vi "Set DeviceData_Status_IO.vi"(8 "error in (no error)":errorcluster, 9 "Trigger Event?":bool, 10 "Device Data":variant=variant(cluster{"DeviceName":string, "COM":refnum<visa-resource-name>, "Status String":string, "Input String":string, "DI Value ":i32}[] []), 11 "IO in":refnum<class "IO.lvclass">) -> (0 "error out":errorcluster, 3 "IO out":refnum<class "IO.lvclass">)   [LabVIEW 2022 SP3, in "IO.lvclass"]
uses:
  IO.lvclass
  IO.lvclass/IO.ctl
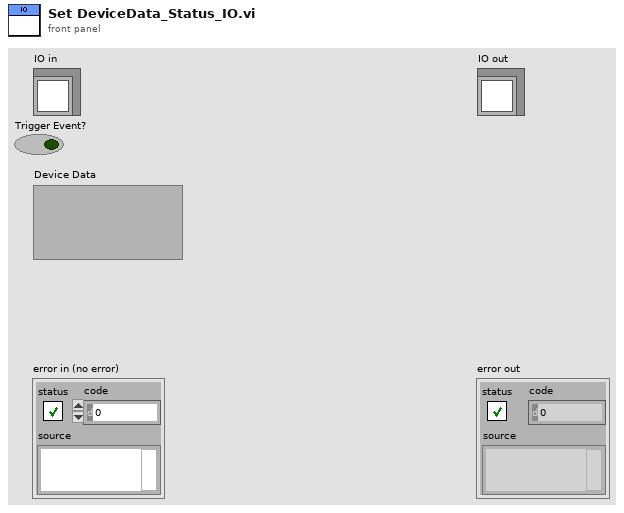
[diagram p1: front panel]
types:
  T1 = typedef "IO.lvclass/Private Data.ctl" = cluster{"UserEvents":T2, "All Dependencies":cluster{"Class References":refnum<class>[], "Class Names":string[]}, "Status":T3}
  T2 = typedef "IO.lvclass/UserEvents.ctl" = cluster{"API Incoming Event":refnum<user-event>, "API Executed Event":refnum<user-event>, "API Return Event":refnum<user-event>, "Status Changed Event":refnum<user-event>}
  T3 = typedef "IO.lvclass/Status Cluster.ctl" = cluster{"Device Data":variant, "Ordered ICP1-DO Channels":T4[], "Ordered ICP2-DI Channels":T5[], "Ordered ICP2-DO Channels":T6[], "Ordered ICP1-AI Channels":T7[], "Ordered ICP1-AO Channels":T8[], "Ordered ICP2-AO Channels":T9[]}
  T4 = typedef "IO.lvclass/ICP1-D0 Channel Names.ctl" = enum16{"None", "Meniscus Pressure Reg PWR - R1", "Meniscus Pressure Reg PWR - R2", "Meniscus Pressure Reg PWR - R3", "Meniscus Pressure Reg PWR - R4", "Meniscus Pressure Reg PWR - R5", "Meniscus Pressure Reg PWR - R6", "Clear Stage Alarm", "Servo ON", "Purge Valve Open - R1", "Purge Valve Open - R2", "Purge Valve Open - R3", "Purge Valve Open - R4", "Purge Valve Open - R5", "Purge Valve Open - R6"}
  T5 = typedef "IO.lvclass/ICP2-DI Channel Names.ctl" = enum16{"None", "SW - Ink Valve - R1", "SW - Ink Valve - R2", "SW - Ink Valve - R3", "SW - Ink Valve - R4", "SW - Ink Valve - R5", "SW - Ink Valve - R6", "SW - COVER INPUT SIDE", "SW - COVER OUTPUT SIDE", "SW - Purge - R1", "SW - Purge - R2", "SW - Purge - R3", "SW - Purge - R4", "SW - Purge - R5", "SW - Purge - R6"}
  T6 = typedef "IO.lvclass/ICP2-DO Channel Names.ctl" = enum16{"None", "Meniscus Valve Open - R1", "Meniscus Valve Open - R2", "Meniscus Valve Open - R3", "Meniscus Valve Open - R4", "Meniscus Valve Open - R5", "Meniscus Valve Open - R6", "Ink Flow Valve Open - R1", "Ink Flow Valve Open - R2", "Ink Flow Valve Open - R3", "Ink Flow Valve Open - R4", "Ink Flow Valve Open - R5", "Ink Flow Valve Open - R6", "SW_LED - Ink Valve - R1", "SW_LED - Ink Valve - R2", "SW_LED - Ink Valve - R3", "Recirc Pump On - R1", "Recirc Pump On - R2", "Recirc Pump On - R3", "Recirc Pump On - R4", "Recirc Pump On - R5", "Recirc Pump On - R6", "SW_LED - Ink Valve - R4", "SW_LED - Ink Valve - R5", "SW_LED - Ink Valve - R6"}
  T7 = typedef "IO.lvclass/ICP1-AI Channel Names.ctl" = enum16{"None", "Meniscus Pressure Read - R1", "Meniscus Pressure Read - R2", "Meniscus Pressure Read - R3", "Meniscus Pressure Read - R4", "Meniscus Pressure Read - R5", "Meniscus Pressure Read - R6", "Meniscus Pressure Set - R1", "Meniscus Pressure Set - R2", "Meniscus Pressure Set - R3", "Meniscus Pressure Set - R4", "Meniscus Pressure Set - R5", "Meniscus Pressure Set - R6"}
  T8 = typedef "IO.lvclass/ICP1-AO Channel Names.ctl" = enum16{"None", "Meniscus Pressure Set - R1", "Meniscus Pressure Set - R2", "Meniscus Pressure Set - R3", "Meniscus Pressure Set - R4", "Meniscus Pressure Set - R5", "Meniscus Pressure Set - R6", "Meniscus Vac Pump Speed"}
  T9 = typedef "IO.lvclass/ICP2-AO Channel Names.ctl" = enum16{"None", "Recirc Pump Flow Set - R1", "Recirc Pump Flow Set - R2", "Recirc Pump Flow Set - R3", "Recirc Pump Flow Set - R4", "Recirc Pump Flow Set - R5", "Recirc Pump Flow Set - R6"}
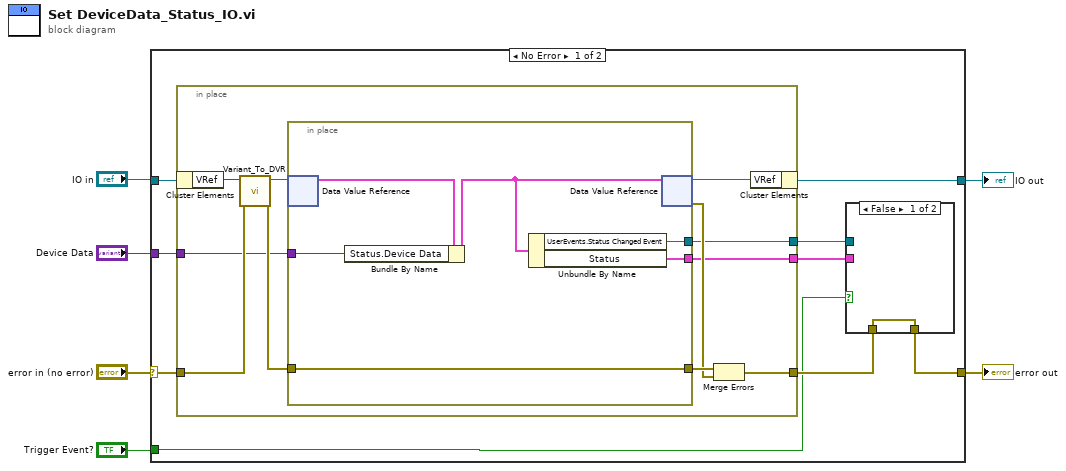
[diagram p0: block diagram]
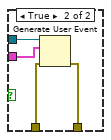
[diagram p2: hidden frame]
diagram:
  n1 = case shown="No Error" "error in (no error)" {
    selector: "error in (no error)" -> [w13 w39]
    tunnel: [w9 w39] -> w4
    tunnel: [w15 w38] -> w3
    tunnel: "IO in" -> [w14 w38]
    tunnel: "Device Data" -> [w12 _]
    tunnel: "Trigger Event?" -> [w7 _]
    frame No Error {
      n2 = in-place {
        in-place-border: w13 -> [w29]
        in-place-border: [w25] -> w10
        in-place-border: w12 -> [w23]
        in-place-border: [w22] -> w11
        in-place-border: [w21] -> w8
        n3 = in-place-cluster #1(w14) -> ("VRef"=w31:variant)
        n4 = call "Variant_To_DVR.vi"("error in (no error)"=w29, "Variant"=w31) -> ("error out"=w28:errorcluster, "DVR"=w30:refnum<data-value>)  [unwired: 8 in]
        n5 = in-place {
          in-place-border: w28 -> [w37]
          in-place-border: [w37] -> w27
          in-place-border: w23 -> [w35]
          in-place-border: [w33] -> w22
          in-place-border: [w32] -> w21
          n6 = in-place-dvr #2(w30) -> (w36:T1)  [unwired: 1 out]
          n7 = Bundle By Name(cluster=w36, "Status.Device Data"=w35) -> (w34:T1)
          n8 = Unbundle By Name(w34) -> ("UserEvents.Status Changed Event"=w33:refnum<user-event>, "Status"=w32:T3)
          n9 = in-place-dvr #2(w34) -> (w24:refnum<data-value>, w26:errorcluster)
        }
        n10 = Merge Errors(w27, w26) -> (w25:errorcluster)
        n11 = in-place-cluster #1("VRef"=w24) -> (w15:refnum<class "IO.lvclass">)
      }
      n12 = case shown="False" w7 {
        tunnel: w11 -> [_ w20]
        tunnel: w10 -> [w16 w19]
        tunnel: [w16 w18] -> w9
        tunnel: w8 -> [_ w17]
        frame False {
        }
        frame True {
          n13 = Generate User Event(user event=w20, event data cluster=w17, error in=w19) -> (error out=w18:errorcluster)  [unwired: 1 in, 1 out]
        }
      }
    }
    frame Error {
    }
  }
  "error out" <- w4
  "IO out" <- w3
